vi "File Load Dialog.vi"(5 "FPGA memory size":T2, 7 "DAC Bits":u16=1 min=1 max=16, 8 "error in (no error)":errorcluster, 10 "CycleAngle?":T3 caption="FPGA simulation angle reference", 11 "Node Ptr":T4 format="%.0x") -> (0 "error out":errorcluster, 2 "Cancelled":bool, 3 "Data":dbl[](array[numeric]))   [LabVIEW 2011, in "Engine Sim System Explorer.lvlib"]
uses:
  Engine Sim System Explorer.lvlib
  TypeDefs/Data Replay Data Selection Method.ctl
  <vilib>/NI Veristand/Custom Device API/Custom Device Item Ref.ctl
  TypeDefs/AngleReference.ctl
  TypeDefs/FPGA Mem Size.ctl
  Data File Loader/Engine Sim File Interface.lvlib
  <vilib>/NI Veristand/Custom Device API/Custom Device API.lvlib
panel:
  in  "DispTwoRotations":bool
  in  "ReverseData":bool
  in  "Missing teeth location (degrees)":dbl=1.0 min=0.0
  in  "DataPlugin":u16(ring)
  out "Loaded samples":i32=1 min=1
  out "Loaded start offset":i32=1 min=0
  in  "Refresh Graph":bool
  in  "Samples":i32=1 min=1
  in  "File start offset":i32=1 min=0
  in  "Data Selection Method":T1
  in  "Channel":u16(ring)
  in  "Selected File":path
  in  "Group":u16(ring)
  in  "Cancel":bool
  in  "OK":bool
  out "Data Graph":waveform(dbl)(graph)
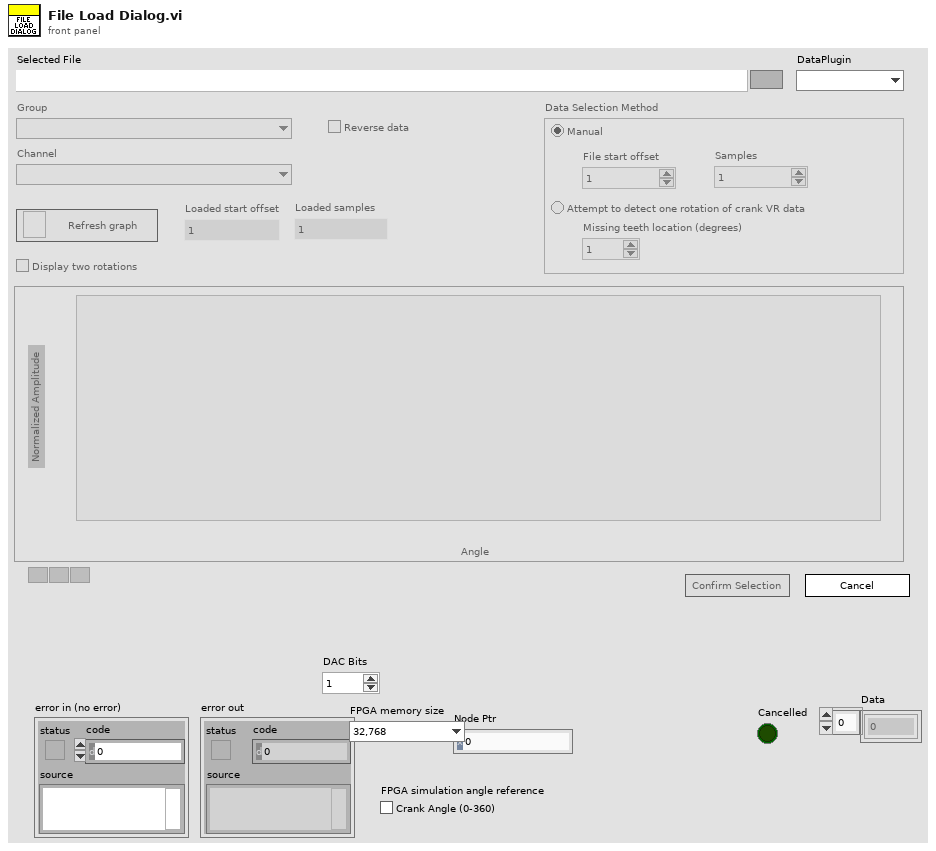
[diagram p1: front panel]
types:
  T1 = typedef "Engine Sim System Explorer.lvlib/Data Replay Data Selection Method.ctl" = enum32{"Manual", "AutoVRCrank"}
  T2 = typedef "Engine Sim System Explorer.lvlib/FPGA Mem Size.ctl" = enum16{"32,768", "16,384", "8,192", "4,096", "2,048", "1024", "512", "256", "128"}
  T3 = typedef "Engine Sim System Explorer.lvlib/AngleReference.ctl" = bool
  T4 = typedef "Custom Device API.lvlib/Custom Device Item Ref.ctl" = u64
  T5 = typedef "Engine Sim System Explorer.lvlib/File Load Dialog.ctl" = cluster{"File":path, "Group":string, "Channel":string, "DataPlugin":string, "MissingTeeth":dbl, "ErrState":string, "File Selected":bool, "Data Selection Method":T1, "Offset":i32, "Length":i32, "DataPlugins Info":T6[], "Controls":refnum<vi>[], "File Ref":refnum<k20>, "Groups":string[], "Channels":string[], "Groups Refs":refnum<k20>[], "Channel Refs":refnum<k20>[], "Cancelled":bool, "CycleAngle?":T3, "FPGA memory size":T2, "DAC Bits":u16, "GroupRef":refnum<k20>, "ChanRef":refnum<k20>, "Data":dbl[], "ReverseData":bool, "DispTwoRotations":bool}
  T6 = typedef "usiPluginInformation.ctl" = cluster{"name":string, "version":string, "type":string, "read-only?":bool, "extensions":string[]}
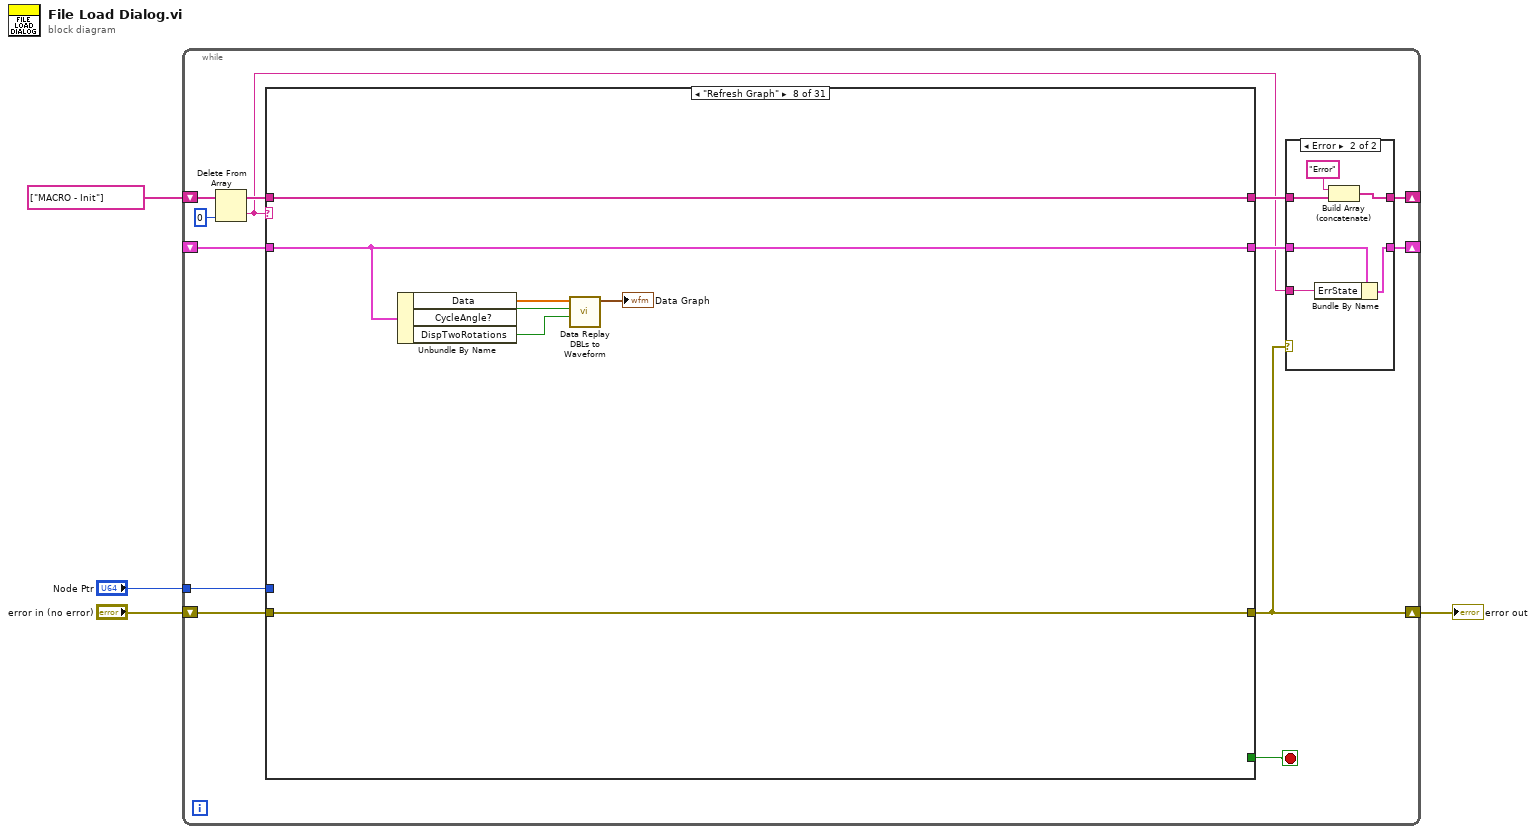
[diagram p0: block diagram]
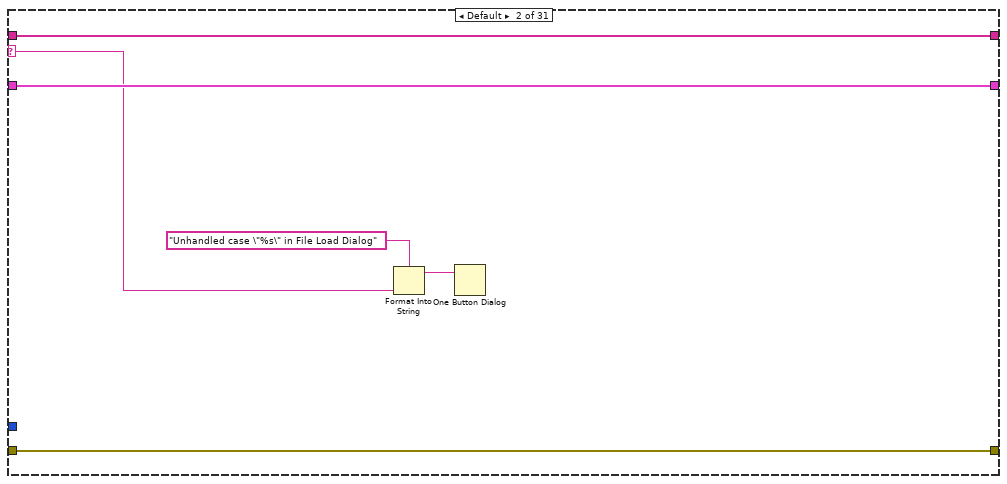
[diagram p4: hidden frame]
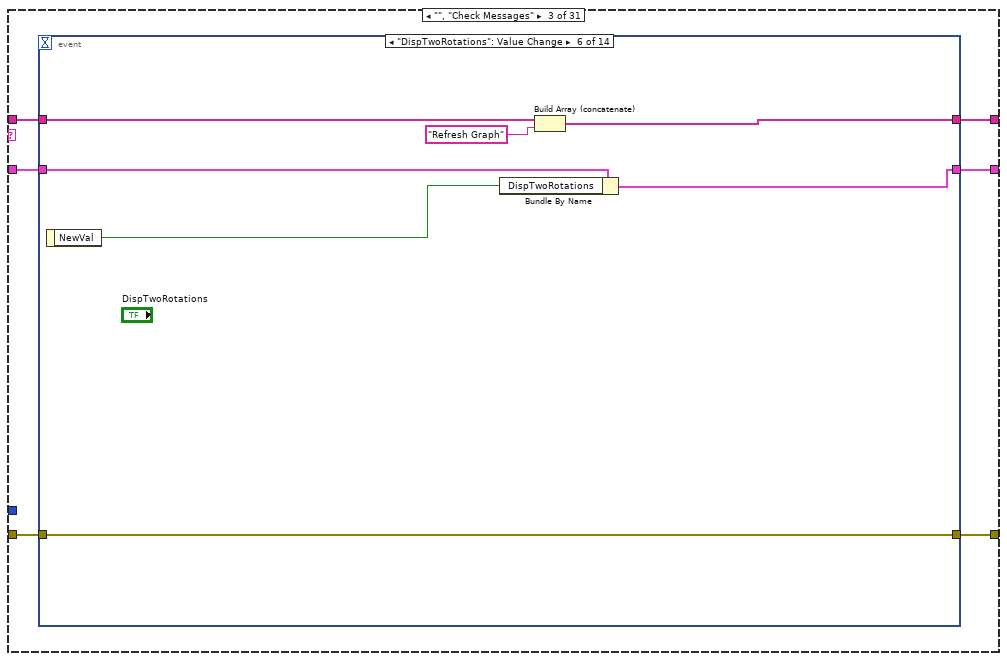
[diagram p5: hidden frame]
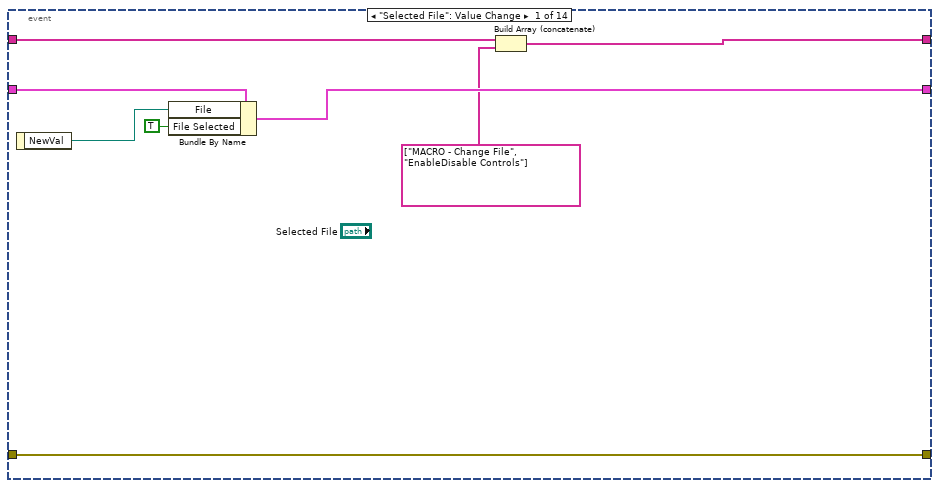
[diagram p6: hidden frame]
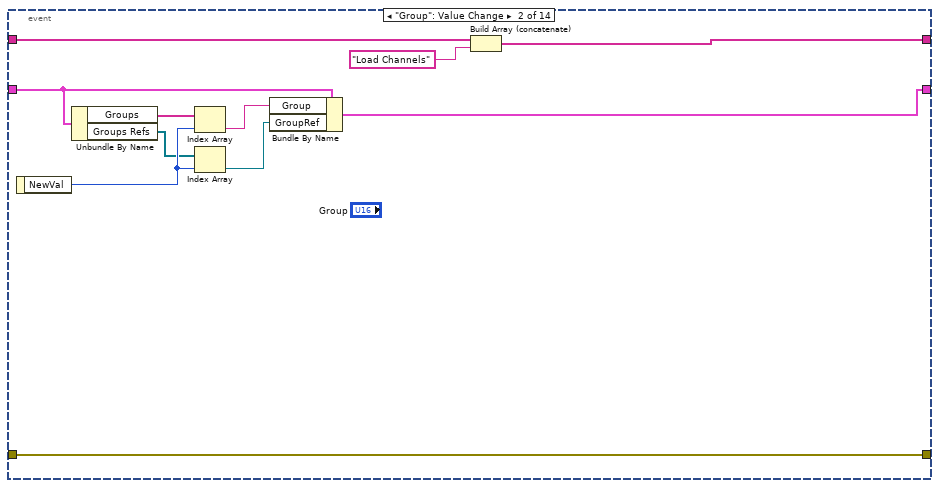
[diagram p7: hidden frame]
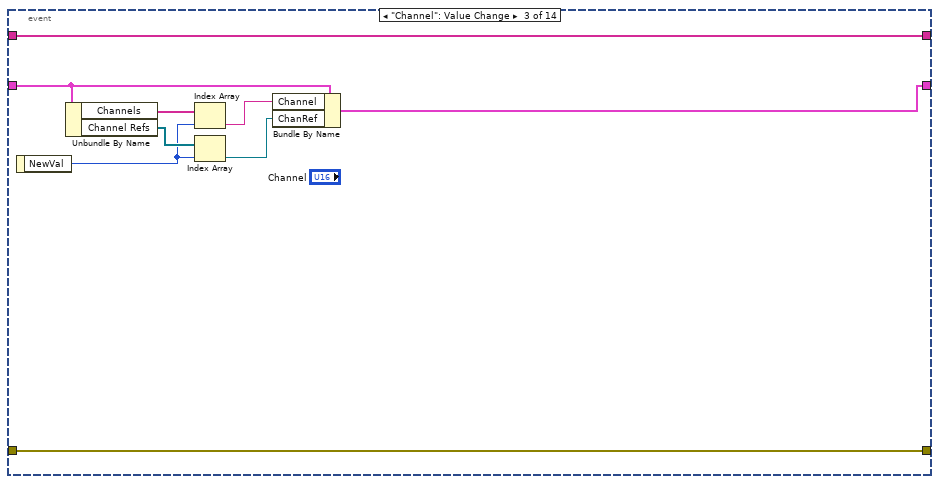
[diagram p8: hidden frame]
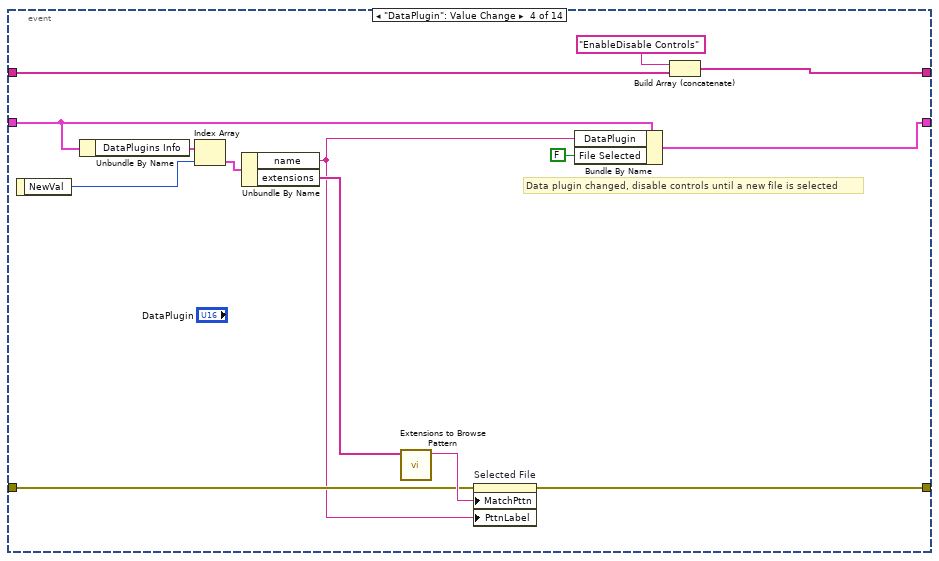
[diagram p9: hidden frame]
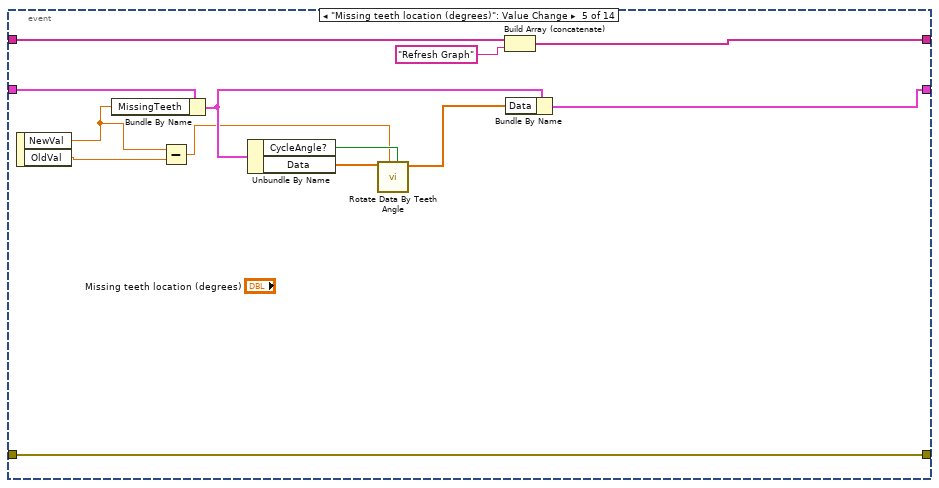
[diagram p10: hidden frame]
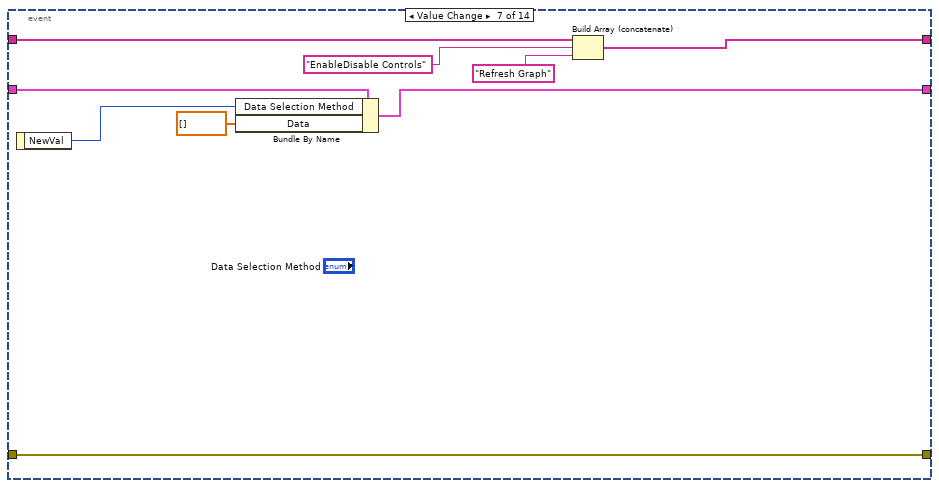
[diagram p11: hidden frame]
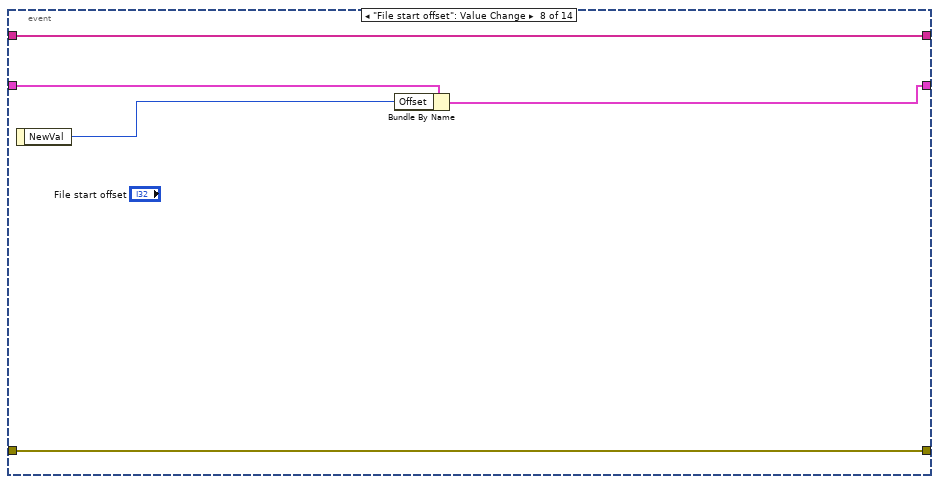
[diagram p12: hidden frame]
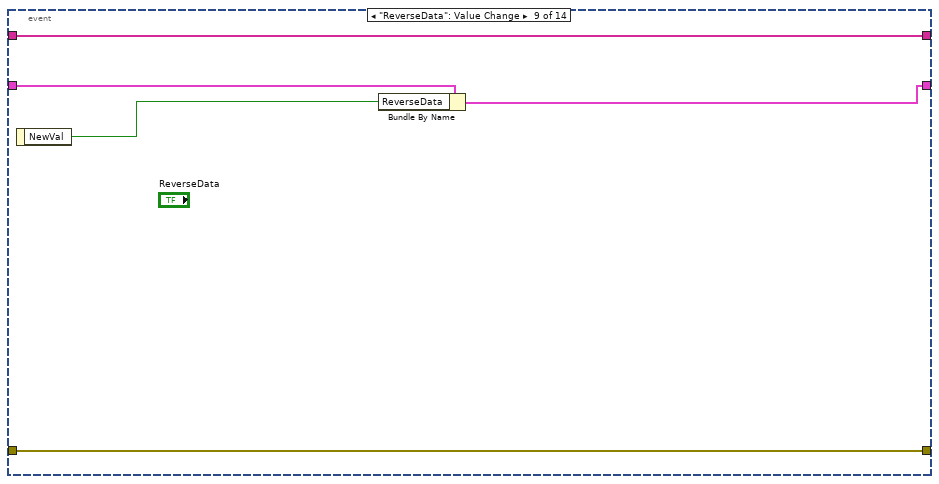
[diagram p13: hidden frame]
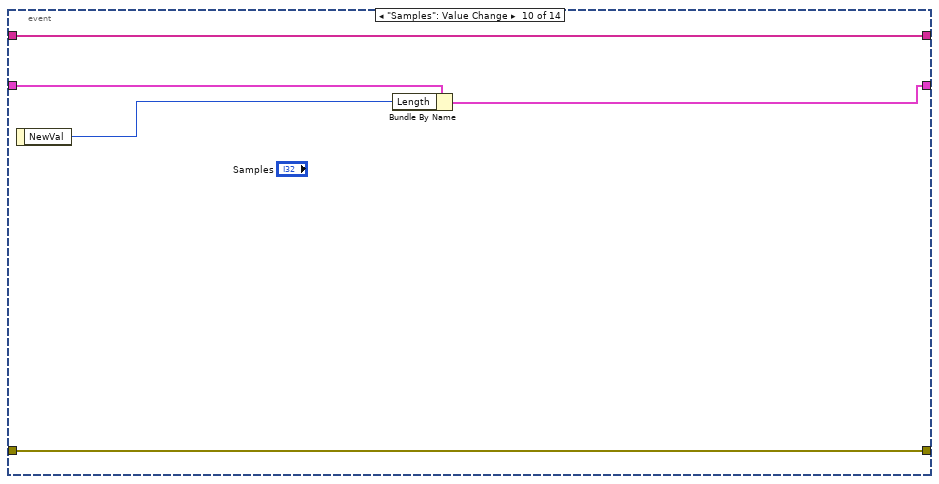
[diagram p14: hidden frame]
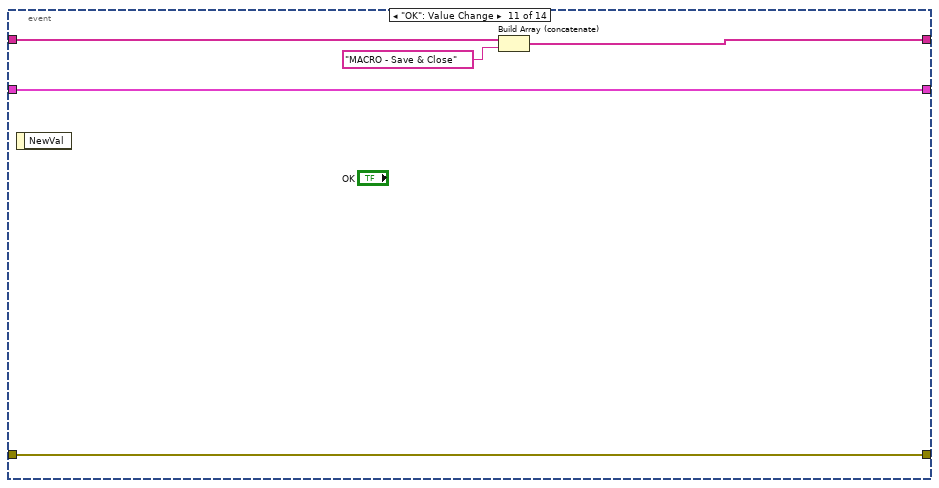
[diagram p15: hidden frame]
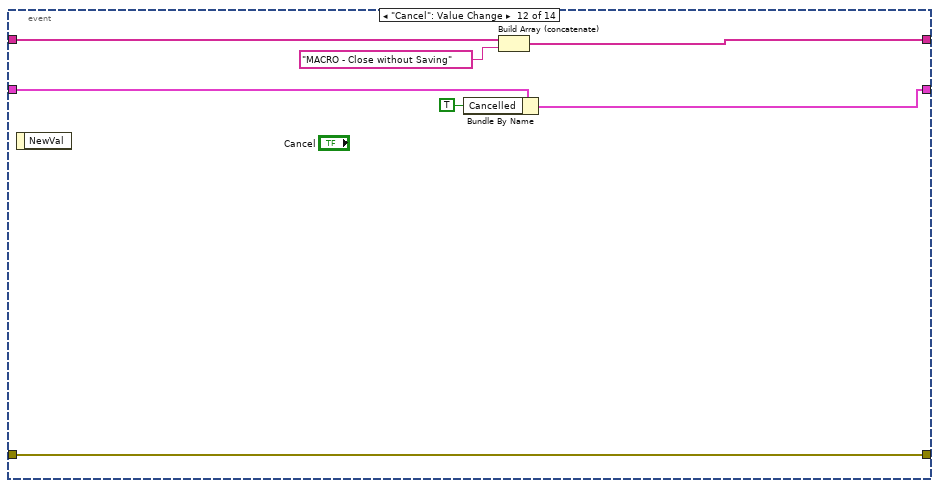
[diagram p16: hidden frame]
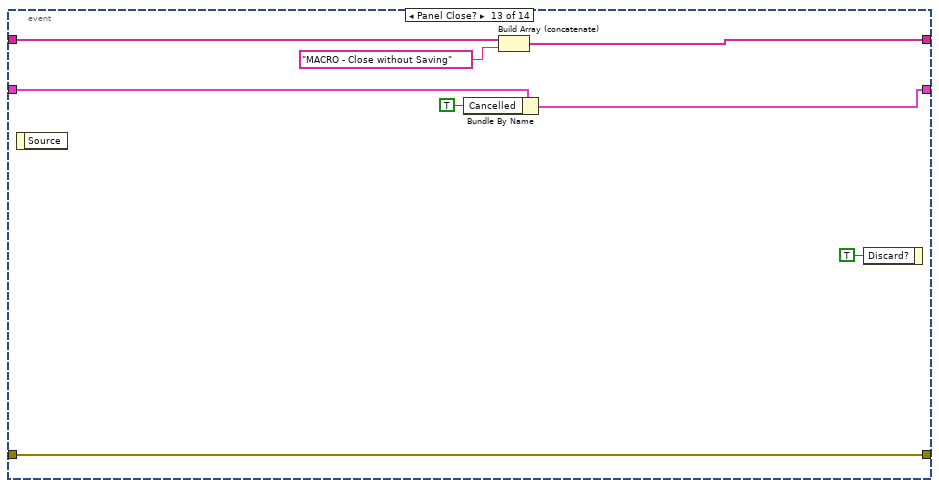
[diagram p17: hidden frame]
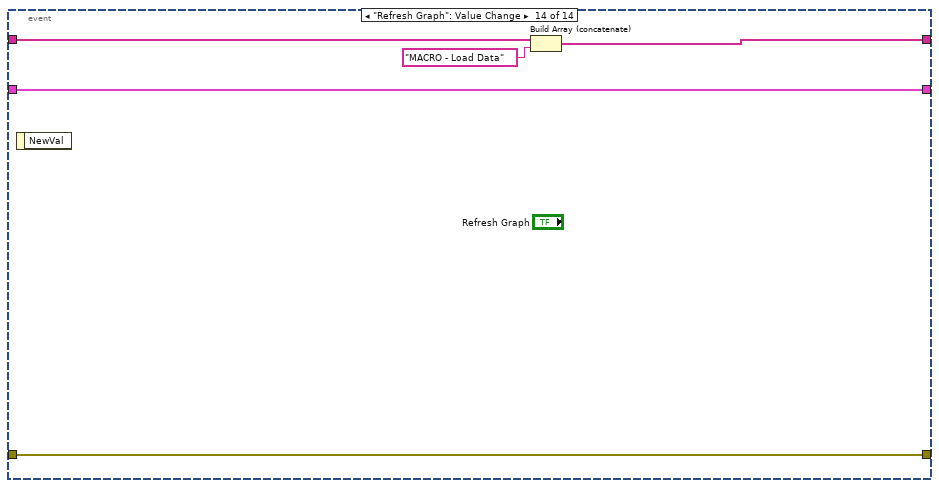
[diagram p18: hidden frame]
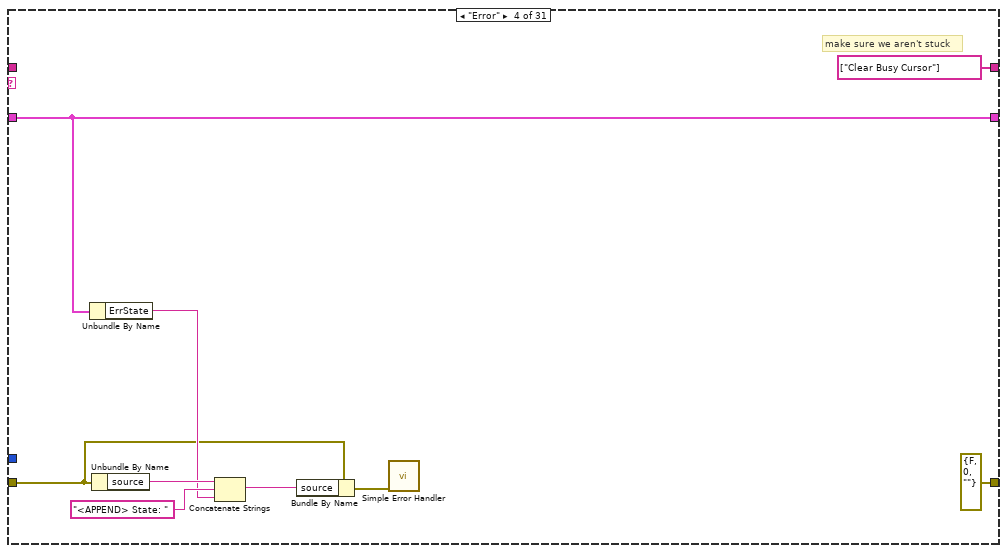
[diagram p19: hidden frame]
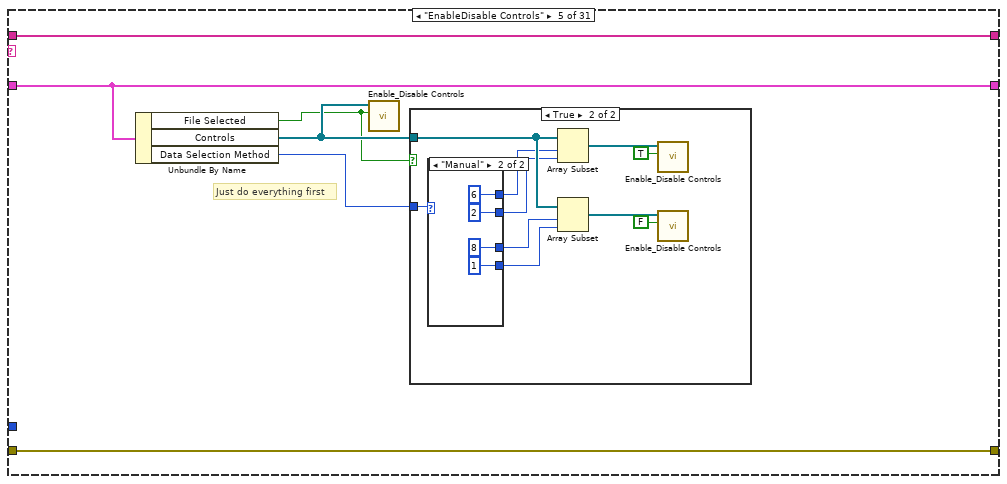
[diagram p20: hidden frame]
diagram:
  n1 = while {
    tunnel: "Node Ptr" -> [w16]
    shift-right: [w12] -> _
    shift-left: string[] ["MACRO - Init"] -> [w15]
    shift-right: [w10] -> _
    shift-left: _ -> [w9]
    shift-right: [w8] -> w1
    shift-left: "error in (no error)" -> [w17]
    stop <- w7 stop-if-true
    n2 = Delete From Array(array=w15, index=0) -> (deleted portion=w5:string, array with subset deleted=w14:string[])  [unwired: 1 in]
    n3 = case shown="\"Refresh Graph\"" w5 {
      selector: w5 -> [_ w29 _ _ _ _ _ _ _ _ _ _ _ _ _ _ _ _ _ _ _ _ _ _ _ _ _ _ _ _ _]
      tunnel: w17 -> [w26 w32 w35 w154 w165 w186 w191 w199 w201 w211 w217 w238 w253 w271 w291 w317 w323 w329 w335 w337 w343 w348 w353 w358 w363 w365 w377 w397 w421 w442 w464]
      tunnel: w16 -> [_ _ _ _ _ _ _ _ _ _ _ _ _ _ _ _ _ w327 _ _ _ _ _ _ _ _ w376 _ _ _ _]
      tunnel: w14 -> [w28 w34 w39 _ w166 w188 w193 w200 w203 w212 w221 w230 w254 w272 w292 w318 w325 w330 w336 w339 w341 w346 w351 w356 w361 w367 w374 w407 w416 w457 w465]
      tunnel: [w28 w34 w40 string[] ["Clear Busy Cursor"] w166 w188 w193 w200 w203 w212 w221 w227 w254 w272 w281 w318 w325 w330 w336 w339 w340 w345 w350 w355 w360 w367 w374 w407 w417 w457 w465] -> w13
      tunnel: [w27 w33 w38 w159 w164 w187 w192 w198 w202 w204 w219 w232 w245 w263 w286 w305 w324 w326 w333 w338 w344 w349 w354 w359 w364 w366 w372 w391 w415 w444 w461] -> w11
      tunnel: [w26 w32 w36 errorcluster {"status"=FALSE, "code"=0, "source"=""} ("error out") w165 w185 w190 w199 w201 w210 w218 w231 w253 w271 w285 w311 w323 w328 w335 w337 w343 w348 w353 w358 w363 w365 w375 w393 w420 w442 w459] -> w8
      tunnel: w9 -> [w27 w33 w37 w159 w164 w187 w192 w198 w202 w206 w220 w233 w250 w268 w287 w307 w324 w326 w333 w338 w344 w349 w354 w359 w364 w366 _ w391 w414 w445 w463]
      tunnel: [_ _ _ _ _ _ _ _ _ _ _ _ _ _ _ _ _ _ TRUE _ _ _ _ _ _ _ _ _ _ _ _] -> w7
      frame "<------------------ System ------------------>" {
      }
      frame Default {
        n4 = Format Into String(format string="Unhandled case \"%s\" in File Load Dialog", w29) -> (resulting string=w30:string)  [unwired: 2 in, 1 out]
        n5 = One Button Dialog(message=w30) -> ()  [unwired: 1 in, 1 out]
      }
      frame "", "Check Messages" {
        n6 = event shown="[5] \"DispTwoRotations\": Value Change" {
          selector: _ -> [_ _ _ _ _ _ _ _ _ _ _ _ _ _]
          dyn-events: _ -> [_ _ _ _ _ _ _ _ _ _ _ _ _ _]
          timeout: _ -> [_ _ _ _ _ _ _ _ _ _ _ _ _ _]
          tunnel: [w42 w53 w63 w70 w87 w99 w106 w116 w121 w126 w128 w135 w143 w148] -> w40
          tunnel: w39 -> [w48 w59 w63 w79 w95 w102 w111 w116 w121 w126 w131 w138 w146 w151]
          tunnel: [w44 w57 w67 w82 w89 w100 w108 w113 w118 w123 w130 w133 w141 w150] -> w38
          tunnel: w37 -> [w47 w56 w66 w81 w93 w97 w109 w115 w120 w125 w130 w137 w145 w150]
          tunnel: [w43 w58 w68 w74 w94 w101 w110 w114 w119 w124 w129 w136 w144 w149] -> w36
          tunnel: w35 -> [w43 w58 w68 w75 w94 w101 w110 w114 w119 w124 w129 w136 w144 w149]
          event "Selected File": Value Change {
            n7 = event-data() -> ("NewVal"=w46:path)  [unwired: 1 in]
            n8 = Bundle By Name(cluster=w47, "File"=w46, "File Selected"=TRUE) -> (w44:T5)
            n9 = Build Array (concatenate)(w48, string[] ["MACRO - Change File", "EnableDisable Controls"]) -> (w42:string[])
          }
          event "Group": Value Change {
            n10 = event-data() -> ("NewVal"=w51:u16)  [unwired: 1 in]
            n11 = Unbundle By Name(w56) -> ("Groups"=w55:string[], "Groups Refs"=w50:refnum<k20>[])
            n12 = Index Array(array=w55, index=w51) -> (element=w54:string)
            n13 = Index Array(array=w50, index=w51) -> (element=w49:refnum<k20>)
            n14 = Bundle By Name(cluster=w56, "Group"=w54, "GroupRef"=w49) -> (w57:T5)
            n15 = Build Array (concatenate)(w59, "Load Channels") -> (w53:string[])
          }
          event "Channel": Value Change {
            n16 = event-data() -> ("NewVal"=w61:u16)  [unwired: 1 in]
            n17 = Unbundle By Name(w66) -> ("Channels"=w65:string[], "Channel Refs"=w62:refnum<k20>[])
            n18 = Index Array(array=w65, index=w61) -> (element=w64:string)
            n19 = Index Array(array=w62, index=w61) -> (element=w60:refnum<k20>)
            n20 = Bundle By Name(cluster=w66, "Channel"=w64, "ChanRef"=w60) -> (w67:T5)
          }
          event "DataPlugin": Value Change {
            # "Data plugin changed, disable controls until a new file is selected"
            n21 = event-data() -> ("NewVal"=w77:u16)  [unwired: 1 in]
            n22 = Unbundle By Name(w81) -> ("DataPlugins Info"=w80:T6[])
            n23 = Index Array(array=w80, index=w77) -> (element=w78:T6)
            n24 = Unbundle By Name(w78) -> ("name"=w72:string, "extensions"=w73:string[])
            n25 = call "Extensions to Browse Pattern.vi"("extensions"=w73) -> ("spreadsheet string"=w76:string)  [unwired: 10 in]
            n26 = property on="Selected File" class="Path"(error in=w75, "MatchPttn"=w76, "PttnLabel"=w72) -> (error out=w74:errorcluster)  [unwired: 1 in, 1 out]
            n27 = Bundle By Name(cluster=w81, "DataPlugin"=w72, "File Selected"=FALSE) -> (w82:T5)
            n28 = Build Array (concatenate)("EnableDisable Controls", w79) -> (w70:string[])
          }
          event "Missing teeth location (degrees)": Value Change {
            n29 = event-data() -> ("NewVal"=w85:dbl, "OldVal"=w84:dbl)  [unwired: 1 in]
            n30 = Bundle By Name(cluster=w93, "MissingTeeth"=w85) -> (w92:T5)
            n31 = Subtract(x=w85, y=w84) -> (x-y=w83:dbl)
            n32 = Unbundle By Name(w92) -> ("CycleAngle?"=w90:T3, "Data"=w91:dbl[])
            n33 = call "Rotate Data By Teeth Angle.vi"("CycleAngle?"=w90, "Missing Tooth Angle"=w83, "One VR Crank Period"=w91) -> ("Rotated to desired angle"=w88:dbl[])  [unwired: 8 in]
            n34 = Build Array (concatenate)(w95, "Refresh Graph") -> (w87:string[])
            n35 = Bundle By Name(cluster=w92, "Data"=w88) -> (w89:T5)
          }
          event "DispTwoRotations": Value Change {
            n36 = event-data() -> ("NewVal"=w96:bool)  [unwired: 1 in]
            n37 = Bundle By Name(cluster=w97, "DispTwoRotations"=w96) -> (w100:T5)
            n38 = Build Array (concatenate)(w102, "Refresh Graph") -> (w99:string[])
          }
          event Value Change {
            n39 = event-data() -> ("NewVal"=w107:T1)  [unwired: 1 in]
            n40 = Bundle By Name(cluster=w109, "Data Selection Method"=w107, "Data"=dbl[] []) -> (w108:T5)
            n41 = Build Array (concatenate)(w111, "EnableDisable Controls", "Refresh Graph") -> (w106:string[])
          }
          event "File start offset": Value Change {
            n42 = event-data() -> ("NewVal"=w112:i32)  [unwired: 1 in]
            n43 = Bundle By Name(cluster=w115, "Offset"=w112) -> (w113:T5)
          }
          event "ReverseData": Value Change {
            n44 = event-data() -> ("NewVal"=w117:bool)  [unwired: 1 in]
            n45 = Bundle By Name(cluster=w120, "ReverseData"=w117) -> (w118:T5)
          }
          event "Samples": Value Change {
            n46 = event-data() -> ("NewVal"=w122:i32)  [unwired: 1 in]
            n47 = Bundle By Name(cluster=w125, "Length"=w122) -> (w123:T5)
          }
          event "OK": Value Change {
            n48 = event-data() -> ()  [unwired: 1 in, 1 out]
            n49 = Build Array (concatenate)(w131, "MACRO - Save & Close") -> (w128:string[])
          }
          event "Cancel": Value Change {
            n50 = event-data() -> ()  [unwired: 1 in, 1 out]
            n51 = Bundle By Name(cluster=w137, "Cancelled"=TRUE) -> (w133:T5)
            n52 = Build Array (concatenate)(w138, "MACRO - Close without Saving") -> (w135:string[])
          }
          event Panel Close? {
            n53 = event-data() -> ()  [unwired: 1 in, 1 out]
            n54 = Bundle By Name(cluster=w145, "Cancelled"=TRUE) -> (w141:T5)
            n55 = Build Array (concatenate)(w146, "MACRO - Close without Saving") -> (w143:string[])
            n56 = event-data("Discard?"=TRUE) -> ()  [unwired: 1 in, 1 out]
          }
          event "Refresh Graph": Value Change {
            n57 = event-data() -> ()  [unwired: 1 in, 1 out]
            n58 = Build Array (concatenate)(w151, "MACRO - Load Data") -> (w148:string[])
          }
        }
      }
      frame "Error" {
        # "make sure we aren't stuck"
        n59 = Unbundle By Name(w159) -> ("ErrState"=w156:string)
        n60 = Unbundle By Name(w154) -> ("source"=w158:string)
        n61 = Concatenate Strings(w158, "<APPEND> State: " ("string"), w156) -> (w155:string)
        n62 = Bundle By Name(cluster=w154, "source"=w155) -> (w153:errorcluster)
        n63 = call <vilib>:"Simple Error Handler.vi"("error in (no error)"=w153) -> ()  [unwired: 4 in, 5 out]
      }
      frame "EnableDisable Controls" {
        # "Just do everything first"
        n64 = Unbundle By Name(w164) -> ("File Selected"=w161:bool, "Controls"=w162:refnum<vi>[], "Data Selection Method"=w163:T1)
        n65 = call "Enable_Disable Controls.vi"("Enable?"=w161, "Controls"=w162) -> ()  [unwired: 10 in]
        n66 = case shown="True" w161 {
          tunnel: w163 -> [_ w176]
          tunnel: w162 -> [_ w175]
          frame False {
          }
          frame True {
            n67 = case shown="\"Manual\"" w176 {
              tunnel: [1 ("length") 2 ("length")] -> w174
              tunnel: [8 ("index") 6 ("index")] -> w173
              tunnel: [6 ("index") 8 ("index")] -> w168
              tunnel: [2 ("length") 1 ("length")] -> w167
              frame "AutoVRCrank" {
              }
              frame "Manual" {
              }
            }
            n68 = Array Subset(array=w175, index=w173, length=w174) -> (w172:refnum<vi>[])
            n69 = Array Subset(array=w175, index=w168, length=w167) -> (w169:refnum<vi>[])
            n70 = call "Enable_Disable Controls.vi"("Enable?"=TRUE, "Controls"=w172) -> ()  [unwired: 10 in]
            n71 = call "Enable_Disable Controls.vi"("Enable?"=FALSE, "Controls"=w169) -> ()  [unwired: 10 in]
          }
        }
      }
      frame "Set Busy Cursor" {
        n72 = call <vilib>:"Set Busy.vi"("error in (no error)"=w186) -> ("error out"=w185:errorcluster)  [unwired: 9 in, 1 out]
      }
      frame "Clear Busy Cursor" {
        n73 = call <vilib>:"Unset Busy.vi"() -> ("error out"=w189:errorcluster)  [unwired: 11 in]
        n74 = Merge Errors(w189, w191) -> (w190:errorcluster)
      }
      frame "Refresh Graph" {
        n75 = Unbundle By Name(w198) -> ("Data"=w197:dbl[], "CycleAngle?"=w196:T3, "DispTwoRotations"=w194:bool)
        n76 = call "Data Replay DBLs to Waveform.vi"("display two rotations? (F)"=w194, "CycleAngle?"=w196, "Data"=w197) -> ("waveform"=→"Data Graph":waveform(dbl))  [unwired: 8 in]
      }
      frame "<------------- File Interaction------------->" {
      }
      frame "Open File" {
        n77 = Unbundle By Name(w206) -> ("File"=w209:path, "DataPlugin"=w208:string)
        n78 = case shown="Default" w208 {
          tunnel: [_ "<allnumericfloat64>yes</allnumericfloat64>"] -> w207
          frame Default {
          }
          frame "CSV" {
            # "Disables auto detect of data type. Forces dbl"
          }
        }
        n79 = call "Open Data File.vi"("error in (no error)"=w211, "Additional parameters"=w207, "Data Plugin"=w208, "File Path"=w209) -> ("error out"=w210:errorcluster, "File Ref"=w205:refnum<k20>)  [unwired: 6 in]
        n80 = Bundle By Name(cluster=w206, "File Ref"=w205) -> (w204:T5)
      }
      frame "Close File" {
        n81 = Unbundle By Name(w220) -> ("File Ref"=w215:refnum<k20>)
        n82 = Not A Number/Path/Refnum?(number/path/refnum=w215) -> (NaN/Path/Refnum?=w214:bool)
        n83 = case shown="False" w214 {
          tunnel: [w224 w225] -> w218
          tunnel: w217 -> [w223 w225]
          tunnel: w215 -> [w222 _]
          frame False {
            n84 = call "Close Data File.vi"("error in (no error)"=w223, "File Ref"=w222) -> ("error out"=w224:errorcluster)  [unwired: 9 in]
          }
          frame True {
          }
        }
        n85 = Bundle By Name(cluster=w220, "File Ref"=refnum<k0> refnum) -> (w219:T5)
      }
      frame "Load Groups" {
        n86 = Unbundle By Name(w233) -> ("File Ref"=w237:refnum<k20>)
        n87 = call "Get Channel Groups.vi"("error in (no error)"=w238, "File Ref in"=w237) -> ("error out"=w236:errorcluster, "Channel Groups"=w235:refnum<k20>[])  [unwired: 7 in, 1 out]
        n88 = for {
          shift-right: [w241] -> w234
          shift-left: w236 -> [w243]
          tunnel: w235 -> [w242] mode=indexing
          tunnel: [w240] -> w229 mode=indexing
          tunnel: [w239] -> w228 mode=indexing
          n89 = call "Get Object Name.vi"("error in (no error)"=w243, "Storage Object in"=w242) -> ("error out"=w241:errorcluster, "Name"=w240:string, "Storage Object out"=w239:refnum<k20>)  [unwired: 7 in]
        }
        n90 = Build Array (concatenate)("Validate Group", w230) -> (w227:string[])
        n91 = property on="Group" class="Ring (strict)"(error in=w234, "Strings []"=w229) -> (error out=w231:errorcluster)  [unwired: 1 in, 1 out]
        n92 = Bundle By Name(cluster=w233, "Groups"=w229, "Groups Refs"=w228) -> (w232:T5)
      }
      frame "Validate Group" {
        n93 = Unbundle By Name(w250) -> ("Groups"=w249:string[], "Group"=w252:string, "Groups Refs"=w247:refnum<k20>[])
        n94 = Search 1D Array(1D array=w249, element=w252) -> (index of element=w251:i32)  [unwired: 1 in]
        n95 = case shown="-1" w251 {
          selector: w251 -> [_ w261]
          tunnel: w250 -> [w259 w260]
          tunnel: w249 -> [w258 _]
          tunnel: [w256 w260] -> w248
          tunnel: [w255 w261] -> w244
          frame -1 {
            w255 = 0
            # "not found. use first"
            n96 = Index Array(array=w258, index=w255) -> (element=w257:string)
            n97 = Bundle By Name(cluster=w259, "Group"=w257) -> (w256:T5)
          }
          frame Default {
            # "Found, set ref"
          }
        }
        n98 = Index Array(array=w247, index=w244) -> (element=w246:refnum<k20>)
        n99 = local write "Group"(w244) -> ()
        n100 = Bundle By Name(cluster=w248, "GroupRef"=w246) -> (w245:T5)
      }
      frame "Validate Channel" {
        n101 = Unbundle By Name(w268) -> ("Channels"=w267:string[], "Channel"=w270:string, "Channel Refs"=w265:refnum<k20>[])
        n102 = Search 1D Array(1D array=w267, element=w270) -> (index of element=w269:i32)  [unwired: 1 in]
        n103 = case shown="-1" w269 {
          selector: w269 -> [_ w279]
          tunnel: w268 -> [w277 w278]
          tunnel: w267 -> [w276 _]
          tunnel: [w274 w278] -> w266
          tunnel: [w273 w279] -> w262
          frame -1 {
            w273 = 0
            # "not found. use first"
            n104 = Index Array(array=w276, index=w273) -> (element=w275:string)
            n105 = Bundle By Name(cluster=w277, "Channel"=w275) -> (w274:T5)
          }
          frame Default {
            # "Found, set ref"
          }
        }
        n106 = Index Array(array=w265, index=w262) -> (element=w264:refnum<k20>)
        n107 = local write "Channel"(w262) -> ()
        n108 = Bundle By Name(cluster=w266, "ChanRef"=w264) -> (w263:T5)
      }
      frame "Load Channels" {
        n109 = Unbundle By Name(w287) -> ("GroupRef"=w284:refnum<k20>)
        n110 = call "Get Channels.vi"("error in (no error)"=w291, "Channel Group in"=w284) -> ("error out"=w290:errorcluster, "Channels"=w289:refnum<k20>[])  [unwired: 7 in, 1 out]
        n111 = for {
          shift-right: [w295] -> w288
          shift-left: w290 -> [w297]
          tunnel: w289 -> [w296] mode=indexing
          tunnel: [w294] -> w283 mode=indexing
          tunnel: [w293] -> w282 mode=indexing
          n112 = call "Get Object Name.vi"("error in (no error)"=w297, "Storage Object in"=w296) -> ("error out"=w295:errorcluster, "Name"=w294:string, "Storage Object out"=w293:refnum<k20>)  [unwired: 7 in]
        }
        n113 = Build Array (concatenate)("Validate Channel", w292) -> (w281:string[])
        n114 = Bundle By Name(cluster=w287, "Channels"=w283, "Channel Refs"=w282) -> (w286:T5)
        n115 = property on="Channel" class="Ring (strict)"(error in=w288, "Strings []"=w283) -> (error out=w285:errorcluster)  [unwired: 1 in, 1 out]
      }
      frame "Load Data" {
        n116 = Unbundle By Name(w307) -> ("CycleAngle?"=w308:T3, "MissingTeeth"=w309:dbl, "ReverseData"=w298:bool, "ChanRef"=w314:refnum<k20>, "Offset"=w312:i32, "Length"=w313:i32, "Data Selection Method"=w300:T1, "FPGA memory size"=w316:T2)
        n117 = call "Memory Size Enum to Numeric.vi"("error in (no error)"=w317, "FPGA Memory Size"=w316) -> ("error out"=w315:errorcluster, "Numeric"=w303:i32)  [unwired: 8 in]
        n118 = case shown="\"AutoVRCrank\"" w300 {
          tunnel: [w320 0 ("Count (0: Read All)")] -> w310
          tunnel: [w319 0 ("index")] -> w299
          tunnel: w313 -> [w320 _]
          tunnel: w312 -> [w319 _]
          frame "Manual", Default {
          }
          frame "AutoVRCrank" {
          }
        }
        n119 = call "Get Channel Data.vi"("error in"=w315, "Count (0: Read All)"=w310, "index"=w299, "Channel in"=w314) -> ("error out"=w311:errorcluster, "Signal"=w304:dbl[])  [unwired: 5 in, 1 out]
        n120 = call "Select Data Subset From Loaded Data.vi"("CycleAngle?"=w308, "Memory Size as number"=w303, "MissingTeeth"=w309, "ReverseData"=w298, "Offset"=w299, "Data Selection Method"=w300, "Signal"=w304) -> ("Selected Length"=→"Loaded samples":i32, "Selected Offset"=→"Loaded start offset":i32, "Resampled Data"=w306:dbl[])  [unwired: 2 in]
        n121 = Bundle By Name(cluster=w307, "Data"=w306) -> (w305:T5)
      }
      frame "<------------------ Shut Down ------------------>" {
      }
      frame "Save Data" {
        n122 = call "Save File Load Dialog Data.vi"("error in (no error)"=w329, "FileDialog"=w326, "Node Ptr"=w327) -> ("error out"=w328:errorcluster)  [unwired: 8 in]
      }
      frame "Exit" {
        n123 = Unbundle By Name(w333) -> ("Cancelled"=→"Cancelled":bool, "Data"=→"Data":dbl[])
      }
      frame "<------------------ Macros ------------------>" {
      }
      frame "MACRO - Init" {
        n124 = Build Array (concatenate)(string[] ["Set Busy Cursor", "Init Data", "Get DataPlugin List", "Validate File Existis", "Get Refs", "Init UI", "EnableDisable Controls", "Clear Busy Cursor"], w341) -> (w340:string[])
      }
      frame "MACRO - Save & Close" {
        n125 = Build Array (concatenate)(string[] ["Close File", "Save Data", "Exit"], w346) -> (w345:string[])
      }
      frame "MACRO - Close without Saving" {
        n126 = Build Array (concatenate)(string[] ["Close File", "Exit"], w351) -> (w350:string[])
      }
      frame "MACRO - Change File" {
        n127 = Build Array (concatenate)(string[] ["Set Busy Cursor", "Close File", "Open File", "Load Groups", "Load Channels", "Clear Busy Cursor"], w356) -> (w355:string[])
      }
      frame "MACRO - Load Data" {
        n128 = Build Array (concatenate)(string[] ["Set Busy Cursor", "Load Data", "Refresh Graph", "Clear Busy Cursor"], w361) -> (w360:string[])
      }
      frame "<------------------ Initialization ------------------>" {
      }
      frame "Init Data" {
        # "Clear graph"
        n129 = call "Init File Load Dialog Data.vi"("error in (no error)"=w377, "Node Ptr"=w376) -> ("error out"=w375:errorcluster, "FileDialog"=w373:T5)  [unwired: 8 in]
        n130 = Bundle By Name(cluster=w373, "CycleAngle?"="CycleAngle?", "FPGA memory size"="FPGA memory size", "DAC Bits"="DAC Bits") -> (w372:T5)
        n131 = local write "Data Graph"(waveform(dbl) {"t0"=timestamp(0 s since 1904-01-01), "dt"=1.0, "Y"=[]} ("Data Graph")) -> ()
      }
      frame "Init UI" {
        # "None of these are user controls"
        n132 = Unbundle By Name(w391) -> ("File"=w394:path, "MissingTeeth"=w406:dbl, "Data Selection Method"=w405:T1, "Offset"=w404:i32, "Length"=w403:i32, "ReverseData"=w378:bool, "DataPlugins Info"=w402:T6[], "DataPlugin"=w395:string)
        n133 = for {
          tunnel: w402 -> [w413] mode=indexing
          tunnel: [w412] -> w401 mode=indexing
          tunnel: [w410] -> w400 mode=indexing
          n134 = Unbundle By Name(w413) -> ("name"=w412:string, "extensions"=w411:string[])
          n135 = Bundle("extensions"=w411) -> (w410:cluster{"extensions":string[]})  [unwired: 1 in]
        }
        n136 = local write "Missing teeth location (degrees)"(w406) -> ()
        n137 = local write "Data Selection Method"(w405) -> ()
        n138 = local write "File start offset"(w404) -> ()
        n139 = local write "ReverseData"(w378) -> ()
        n140 = local write "Selected File"(w394) -> ()
        n141 = local write "Samples"(w403) -> ()
        n142 = Search 1D Array(1D array=w401, element=w395) -> (index of element=w392:i32)  [unwired: 1 in]
        n143 = Index Array(array=w400, index=w392) -> (element=w399:cluster{"extensions":string[]})
        n144 = local write "DataPlugin"(w392) -> ()
        n145 = Unbundle(w399) -> ("extensions"=w398:string[])
        n146 = call "Extensions to Browse Pattern.vi"("extensions"=w398) -> ("spreadsheet string"=w396:string)  [unwired: 10 in]
        n147 = control-ref of="Cancelled"() -> (w389:refnum<vi>)
        n148 = control-ref of="CycleAngle?"() -> (w388:refnum<vi>)
        n149 = control-ref of="error in (no error)"() -> (w381:refnum<vi>)
        n150 = control-ref of="error out"() -> (w380:refnum<vi>)
        n151 = control-ref of="DAC Bits"() -> (w387:refnum<vi>)
        n152 = control-ref of="Loaded samples"() -> (w384:refnum<vi>)
        n153 = control-ref of="Loaded start offset"() -> (w383:refnum<vi>)
        n154 = control-ref of="Node Ptr"() -> (w382:refnum<vi>)
        n155 = control-ref of="FPGA memory size"() -> (w385:refnum<vi>)
        n156 = control-ref of="Data"() -> (w386:refnum<vi>)
        n157 = property on="Selected File" class="Path"(error in=w397, "MatchPttn"=w396, "PttnLabel"=w395) -> (error out=w393:errorcluster)  [unwired: 1 in, 1 out]
        n158 = Build Array(w389, w388, w387, w386, w385, w384, w383, w382, w381, w380) -> (w379:refnum<vi>[])
        n159 = for {
          tunnel: TRUE ("Skip When Tabbing") -> [w409]
          tunnel: w379 -> [w408] mode=indexing
          n160 = property on="Property Node" class="Ctl"(reference=w408, "SkipTabbing"=w409) -> ()  [unwired: 1 in, 2 out]
        }
      }
      frame "Validate File Existis" {
        n161 = Unbundle By Name(w414) -> ("File"=w419:path, "File Selected"=w418:bool)
        n162 = case shown="False" w418 {
          tunnel: w421 -> [w424 w435]
          tunnel: [w424 w434] -> w420
          tunnel: w419 -> [_ w425]
          tunnel: [w423 w430] -> w417
          tunnel: w416 -> [w423 w431]
          tunnel: [w422 w428] -> w415
          tunnel: w414 -> [w422 w429]
          frame False {
          }
          frame True {
            n163 = call <vilib>:"Check if File or Folder Exists.vi"("error in (no error)"=w435, "path"=w425) -> ("error out"=w434:errorcluster, "file or folder exists?"=w427:bool)  [unwired: 7 in, 1 out]
            n164 = Select(t=w425, s=w427, f=path "") -> (s? t:f=w432:path)
            n165 = case shown="True" w427 {
              tunnel: "MACRO - Change File" -> [_ w439]
              tunnel: w431 -> [w436 w438]
              tunnel: [w436 w437] -> w430
              frame False {
              }
              frame True {
                n166 = Build Array (concatenate)(w439, w438) -> (w437:string[])
              }
            }
            n167 = Bundle By Name(cluster=w429, "File Selected"=w427, "File"=w432) -> (w428:T5)
          }
        }
      }
      frame "Get Refs" {
        n168 = control-ref of="Data Selection Method"() -> (w451:refnum<vi>)
        n169 = control-ref of="Data Graph"() -> (w446:refnum<vi>)
        n170 = control-ref of="ReverseData"() -> (w441:refnum<vi>)
        n171 = control-ref of="DispTwoRotations"() -> (w440:refnum<vi>)
        n172 = control-ref of="File start offset"() -> (w450:refnum<vi>)
        n173 = control-ref of="Refresh Graph"() -> (w454:refnum<vi>)
        n174 = control-ref of="OK"() -> (w447:refnum<vi>)
        n175 = control-ref of="Loaded start offset"() -> (w453:refnum<vi>)
        n176 = control-ref of="Loaded samples"() -> (w452:refnum<vi>)
        n177 = control-ref of="Samples"() -> (w449:refnum<vi>)
        n178 = control-ref of="Missing teeth location (degrees)"() -> (w448:refnum<vi>)
        n179 = control-ref of="Group"() -> (w456:refnum<vi>)
        n180 = control-ref of="Channel"() -> (w455:refnum<vi>)
        n181 = Build Array(w456, w455, w454, w453, w452, w451, w450, w449, w448, w447, w446, w441, w440) -> (w443:refnum<vi>[])
        n182 = Bundle By Name(cluster=w445, "Controls"=w443) -> (w444:T5)
      }
      frame "Get DataPlugin List" {
        n183 = call <vilib>:"List DataPlugins.vi"("error in (no error)"=w464) -> ("DataPlugin information"=w460:T6[], "error out"=w462:errorcluster)  [unwired: 13 in]
        n184 = for {
          tunnel: w460 -> [w467] mode=indexing
          tunnel: [w466] -> w458 mode=indexing
          n185 = Unbundle By Name(w467) -> ("name"=w466:string)
        }
        n186 = Bundle By Name(cluster=w463, "DataPlugins Info"=w460) -> (w461:T5)
        n187 = property on="DataPlugin" class="Ring (strict)"(error in=w462, "Strings []"=w458) -> (error out=w459:errorcluster)  [unwired: 1 in, 1 out]
      }
    }
    n188 = case shown="Error" w8 {
      tunnel: w13 -> [w18 w25]
      tunnel: [w18 w23] -> w12
      tunnel: w11 -> [w19 w22]
      tunnel: [w19 w21] -> w10
      tunnel: w5 -> [_ w20]
      frame No Error {
      }
      frame Error {
        n189 = Bundle By Name(cluster=w22, "ErrState"=w20) -> (w21:T5)
        n190 = Build Array (concatenate)("Error", w25) -> (w23:string[])
      }
    }
  }
  "error out" <- w1
